vi "aw_WRDCluster_8acel_prueba.vi"(0 "ds_id":string, 1 "ds_ss":T1(array[cluster]), 5 "ds_st":dbl, 7 "g_ts":dbl, 9 "g_st":dbl, 11 "ds_ts":dbl) -> (4 "output cluster":T2)   [LabVIEW 2015]
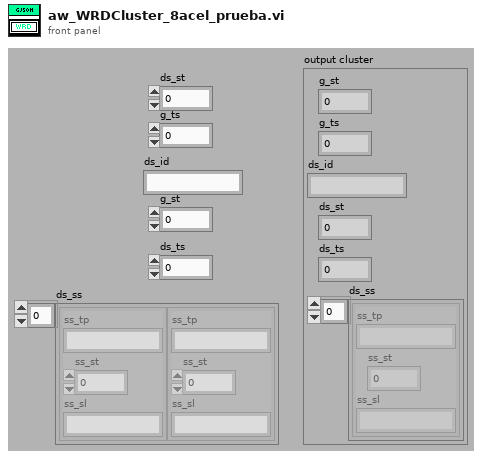
[diagram p1: front panel]
types:
  T1 = cluster{"ss_tp":string, "ss_st":dbl, "ss_sl":string}[]
  T2 = cluster{"g_st":dbl, "g_ts":dbl, "ds_id":string, "ds_st":dbl, "ds_ts":dbl, "ds_ss":cluster{"ss_tp":string, "ss_st":dbl, "ss_sl":string}[]}
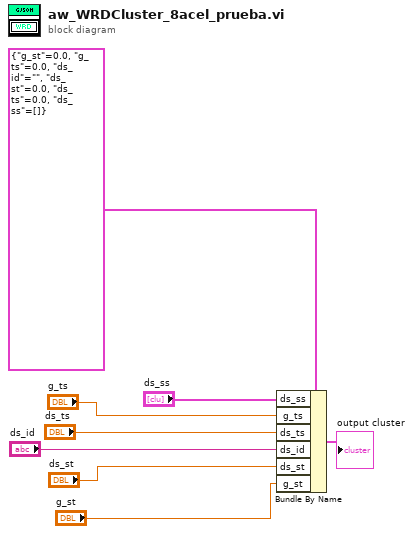
[diagram p0: block diagram]
diagram:
  n1 = Bundle By Name(cluster=T2 {"g_st"=0.0, "g_ts"=0.0, "ds_id"="", "ds_st"=0.0, "ds_ts"=0.0, "ds_ss"=[]}, "ds_ss"="ds_ss", "g_ts"="g_ts", "ds_ts"="ds_ts", "ds_id"="ds_id", "ds_st"="ds_st", "g_st"="g_st") -> (→"output cluster":T2)
